vi "Write Alarm - Message.vi"(8 "error in (no error)":errorcluster, 10 "alarm message":string, 11 "NT Base in":refnum<class "NT Base.lvclass">) -> (0 "error out":errorcluster, 3 "NT Base out":refnum<class "NT Base.lvclass">)   [LabVIEW 2020, in "PV Access.lvlib" / "PV Data.lvlib" / "NT Base.lvclass"]
uses:
  NT Base.lvclass
  NT Base.lvclass/NT Base.ctl
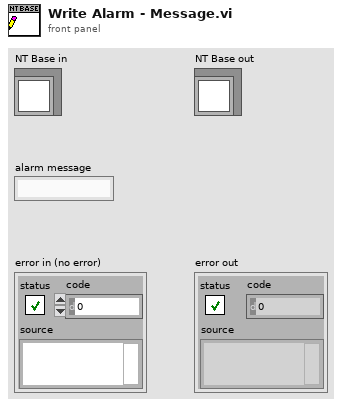
[diagram p1: front panel]
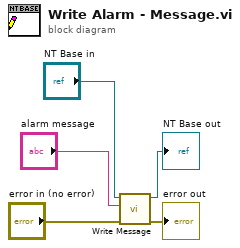
[diagram p0: block diagram]
diagram:
  n1 = call-dynamic "Write Message.vi"("error in"="error in (no error)", "message"="alarm message", "Has Alarm in"="NT Base in") -> ("error out"=→"error out":errorcluster, "Has Alarm out"=→"NT Base out":refnum<class "NT Base.lvclass">)  [unwired: 7 in]
